vi "相机写曝光时间.vi"(9 "选择相机和拍照对象":T1, 11 "Session in":T2 caption="Session Out") -> (3 "Session Out":T2)   [LabVIEW 2014]
uses:
  <vilib>/userdefined/High Color/IMAQdx.ctl
  Controls/MsgAction.ctl
  Global.vi
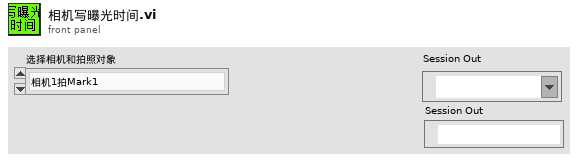
[diagram p1: front panel]
types:
  T1 = typedef "控件-选择相机和拍照对象.ctl" = enum16{"相机1拍Mark1", "相机1拍Mark2", "相机1拍二维码", "相机2"}
  T2 = typedef "IMAQdx.ctl" = refnum<k21>
  T3 = typedef "MsgAction.ctl" = enum16{"初始化", "添加消息", "区分结果添加消息", "清空消息", "获取消息"}
  T4 = typedef "OtherSpec.ctl" = cluster{"其它勾选类规格":T5, "其它数据类规格":T6, "相机名称":T7, "参数":cluster{"Mark1曝光时间":i32, "Mark2曝光时间":i32, "二维码曝光时间":i32}}
  T5 = typedef "其它勾选类规格.ctl" = cluster{"保存图片":bool, "上传设备状态数据":bool, "保存数据":bool, "开机默认开启监控摄像头":bool, "启用mark拍照 ":bool}
  T6 = typedef "其他数据类规格.ctl" = cluster{"相机1像素-毫米换算系数":dbl, "相机2像素-毫米换算系数":dbl, "D盘剩余空间预警(G)":dbl, "视频最长录制时间(秒)":dbl}
  T7 = typedef "相机名称品牌使用状态.ctl" = cluster{"相机1名称":T2, "相机2名称":T2, "Cam1启用":bool, "Cam2启用":bool, "Basler1":bool, "Basler2":bool}
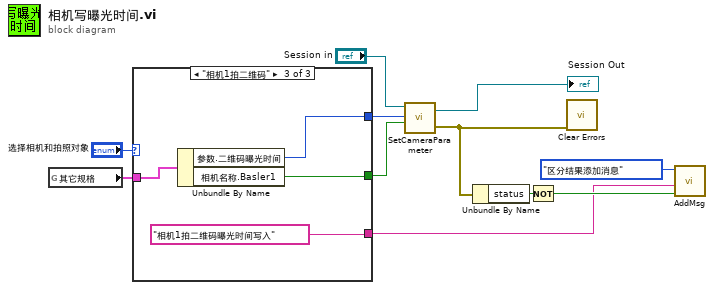
[diagram p0: block diagram]
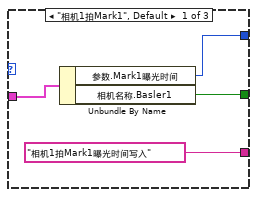
[diagram p2: hidden frame]
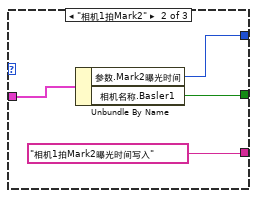
[diagram p3: hidden frame]
diagram:
  n1 = global read "Global.vi" "其它规格"() -> (w9:T4)
  n2 = case shown="\"相机1拍二维码\"" "选择相机和拍照对象" {
    tunnel: [w12 w16 w20] -> w11
    tunnel: w9 -> [w15 w19 w23]
    tunnel: [w14 w18 w22] -> w8
    tunnel: ["相机1拍Mark1曝光时间写入" ("消息显示") "相机1拍Mark2曝光时间写入" ("消息显示") "相机1拍二维码曝光时间写入" ("消息显示")] -> w3
    frame "相机1拍Mark1", Default {
      n3 = Unbundle By Name(w15) -> ("参数.Mark1曝光时间"=w12:i32, "相机名称.Basler1"=w14:bool)
    }
    frame "相机1拍Mark2" {
      n4 = Unbundle By Name(w19) -> ("参数.Mark2曝光时间"=w16:i32, "相机名称.Basler1"=w18:bool)
    }
    frame "相机1拍二维码" {
      n5 = Unbundle By Name(w23) -> ("参数.二维码曝光时间"=w20:i32, "相机名称.Basler1"=w22:bool)
    }
  }
  n6 = call "SetCameraParameter.vi"("相机品牌为Basler?"=w8, "Exposure time"=w11, "Session In"="Session in") -> ("error out"=w4:errorcluster, "Session Out"=→"Session Out":T2)  [unwired: 1 in]
  n7 = Unbundle By Name(w4) -> ("status"=w7:bool)
  n8 = Not(x=w7) -> (.not. x?=w5:bool)
  n9 = call <vilib>:"Clear Errors.vi"("error in (no error)"=w4) -> ()  [unwired: 5 in, 2 out]
  n10 = call "AddMsg.vi"("Result"=w5, "添加消息"=w3, "消息Action"=MsgAction."区分结果添加消息") -> ()  [unwired: 1 in, 1 out]
